vi "ex13.vi"() -> ()   [LabVIEW 2019]
panel:
  out "x+y":dbl
  in  "y":dbl
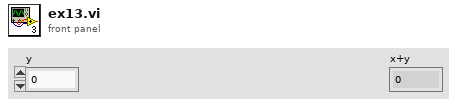
[diagram p1: front panel]
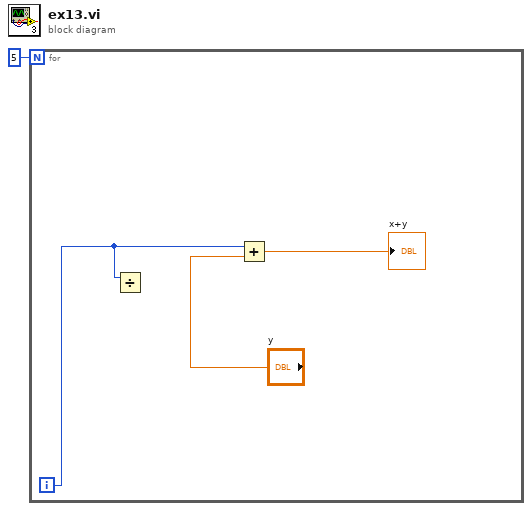
[diagram p0: block diagram]
diagram:
  n1 = for {
    N: 5 -> [_]
    i -> [w2]
    n2 = Divide(x=w2) -> ()  [unwired: 1 in, 1 out]
    n3 = Add(x=w2, y="y") -> (x+y=→"x+y":dbl)
  }
